vi "Echo.vi"   [LabVIEW 2011]
uses:
  CLI Class/CLI.lvclass
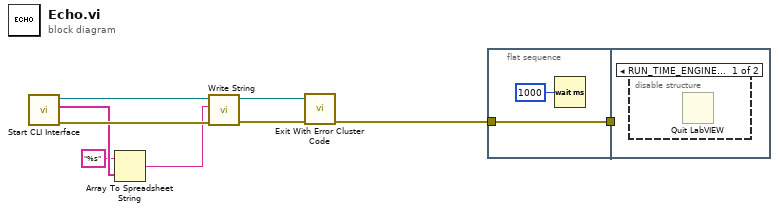
[diagram p0: block diagram]
diagram:
  n1 = call "Start CLI Interface.vi"() -> ("error out"=w5:errorcluster, "Custom Parameters"=w4:string[], "CLI out"=w6:refnum<class "CLI.lvclass">)  [unwired: 8 in, 1 out]
  n2 = Array To Spreadsheet String(array=w4, 3:"%s" ("format string")) -> (spreadsheet string=w2:string)  [unwired: 1 in]
  n3 = call "Write String.vi"("error in (no error)"=w5, "Text to Write"=w2, "CLI in"=w6) -> ("error out"=w8:errorcluster, "CLI out"=w7:refnum<class "CLI.lvclass">)  [unwired: 7 in]
  n4 = call "Exit With Error Cluster Code.vi"("error in (no error)"=w8, "CLI in"=w7) -> ("error out"=w1:errorcluster)  [unwired: 9 in]
  n5 = flat-sequence {
    tunnel: w1 -> [w11]
    tunnel: [w11] -> w9
    tunnel: w9 -> [_]
    frame #0 {
      n6 = Wait (ms)(milliseconds to wait=u32 1000) -> ()  [unwired: 1 out]
    }
    frame #1 {
      n7 = disable-structure shown="RUN_TIME_ENGINE==True" {
        frame condition #0 {
          n8 = Quit LabVIEW() -> ()  [unwired: 1 in]
        }
        frame condition #1 (active) {
        }
      }
    }
  }
